vi "acquiringTank2.vi"() -> ()   [LabVIEW 2012]
uses:
  <vilib>/Platform/TimedLoop/XDataNode/timing_clust.ctl
  <vilib>/Platform/TimedLoop/XDataNode/nitl_modes.ctl
  <vilib>/Platform/TimedLoop/XDataNode/wakeup.ctl
  <vilib>/imath/engines/lvmath2/RunTimeEngine/ErrorHandling/NIMS_Finalize Error.vi
  <vilib>/imath/engines/lvmath2/RunTimeEngine/BuiltInFunctions/size/NIMS_I32=size(GM,I32).vi
  <instcachedir>/0/NIMS_I32=size(GM,I32)_AF436776B5724EA8A5CFD6FACA63D3D9.lvgen/NIMS_I32=size(GM,I32)_AF436776B5724EA8A5CFD6FACA63D3D9_004.vi
  <vilib>/imathl/engines/lvmath/Functions/Error Handling/Create Error.vi
  <vilib>/imath/engines/lvmath2/RunTimeEngine/VariableToken/Read/NIMS_Get Elements - SorM(_,_) - Check - Check.vi
  <instcachedir>/0/NIMS_Get Elements - SorM(_,_) - Check - Check_3492346BAECA4EC09E2016EA7EC0034B.lvgen/NIMS_Get Elements - SorM(_,_) - Check - Check_3492346BAECA4EC09E2016EA7EC0034B_001.vi
  <vilib>/imath/engines/lvmath2/RunTimeEngine/NodeEndStatement/NIMS_NodeEndStatement_Output.vi
  <instcachedir>/0/NIMS_NodeEndStatement_Output_53EC0D466D134D7ABD903AC30B43404B.lvgen/NIMS_NodeEndStatement_Output_53EC0D466D134D7ABD903AC30B43404B_001.vi
  <instcachedir>/0/NIMS_NodeEndStatement_Output_53EC0D466D134D7ABD903AC30B43404B.lvgen/NIMS_NodeEndStatement_Output_53EC0D466D134D7ABD903AC30B43404B_013.vi
  <vilib>/Platform/TimedLoop/XDataNode/XDataNode.xnode
  <vilib>/Platform/TimedLoop/XDataNode/XDNodeRunTimeDep.lvlib
panel:
  out "Find":bool
  out "Numeric":dbl
  out "Angle":dbl(knob) scale=-35.0..35.0
  out "isNotGetten":bool
  out "Angle":dbl[][](array[numeric])
  in  "Stop (F)":bool
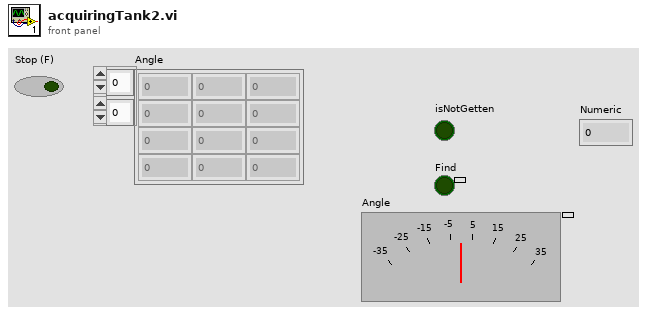
[diagram p1: front panel]
types:
  T1 = typedef "XDNodeRunTimeDep.lvlib/timing_clust.ctl" = cluster{"Expected End [f-1]":u64, "Actual End [f-1]":u64, "Finished Late? [f-1]":bool, "Expected End [i-1]":u64, "Actual End [i-1]":u64, "Finished Late? [i-1]":bool, "Expected Start [i]":u64, "Actual Start [i]":u64, "Expected Start [f]":u64, "Actual Start [f]":u64, "Source Name":string, "Structure Name":string, "Period":i64, "Deadline":i64, "Offset":i64, "Start":i64, "Priority":i32, "Timeout":i32, "Mode":T2, "Wakeup Reason":T3, "Error":errorcluster, "Source Type":string, "Secondary Source Type":string, "Global End Time":u64, "Global Start Time":u64, "Frame Duration":u64, "Iteration Duration":u64, "Assigned CPU":i32, "I/O Scan Engine Mode":u32}
  T2 = typedef "XDNodeRunTimeDep.lvlib/nitl_modes.ctl" = enum32{"No Change", "Process missed periods, maintain original phase", "Discard missed periods, maintain original phase", "Process missed periods, ignore original phase", "Discard missed periods, ignore original phase"}
  T3 = typedef "XDNodeRunTimeDep.lvlib/wakeup.ctl" = enum32{"Normal", "Aborted", "Asynchronous wakeup", "Timing source error", "Timed loop error", "Timeout"}
  T4 = typedef "IMAQ Image.ctl" = refnum<image>
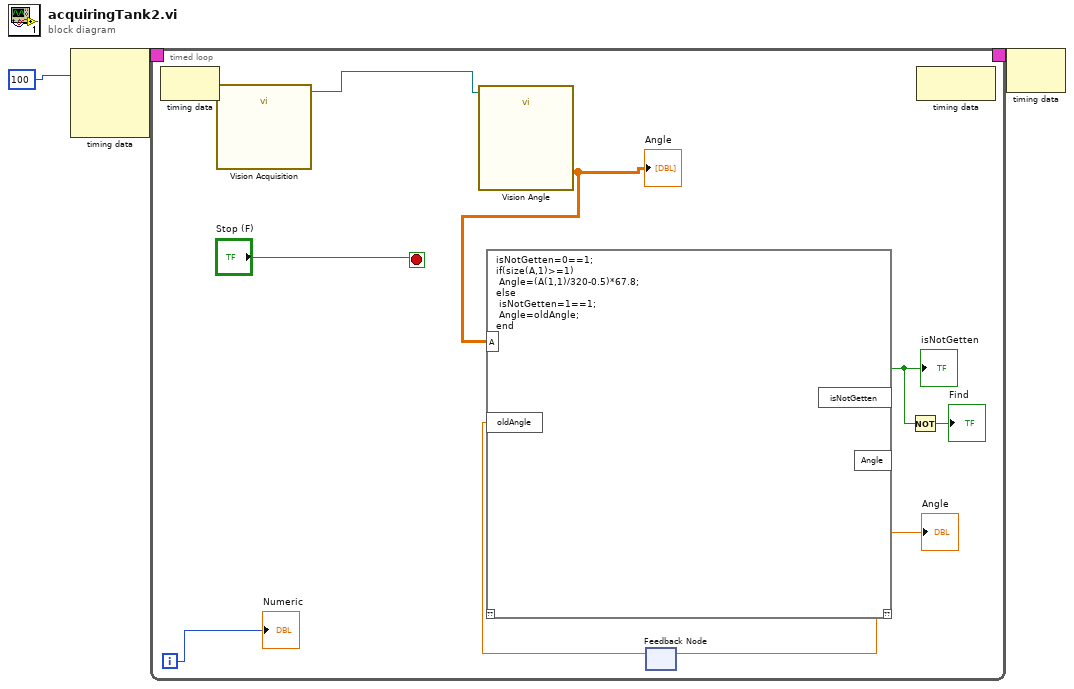
[diagram p0: block diagram]
diagram:
  n1 = node-c288(100) -> (w3:T1)  [unwired: 3 in]
  n2 = timed-loop {
    timing: w3 -> [_]
    timing-out: [_] -> w2
    i -> [w6]
    stop <- "Stop (F)" stop-if-true
    n3 = node-c288() -> ()  [unwired: 1 in, 1 out]
    n4 = call "Vision Acquisition"() -> ("Image Out"=w11:T4)  [unwired: 25 in, 2 out]
    n5 = call "Vision Angle"("Image In"=w11) -> ("Particle Measurements (Pixels) (Particle Analysis 1)"=w9:dbl[][])  [unwired: 23 in, 3 out]
    "Angle" <- w9
    n6 = feedback #1() -> (w8:dbl)  [unwired: 1 in]
    n7 = mathscript code="isNotGetten=0==1;\nif(size(A,1)>=1)\n Angle=(A(1,1)/320-0.5)*67.8;\nelse\n isNotGetten=1==1;\n Angle=oldAngle;\nend"("A"=w9, "oldAngle"=w8) -> ("Angle"=w7:dbl, "isNotGetten"=w5:bool)  [unwired: 1 in, 1 out]
    "Angle" <- w7
    "isNotGetten" <- w5
    n8 = feedback-in #1(w7) -> ()
    n9 = Not(x=w5) -> (.not. x?=→"Find":bool)
    n10 = node-c288() -> ()  [unwired: 1 in, 1 out]
    "Numeric" <- w6
  }
  n11 = node-c288(w2) -> ()  [unwired: 1 out]
